vi "Editor UI.vi"(10 "Close Event":refnum<user-event>, 11 "Simulated Waveform in":refnum<class "Simulated Waveform.lvclass">) -> ()   [LabVIEW 2020, in "Simulated Waveform.lvlib" / "Simulated Waveform.lvclass"]
uses:
  Simulated Waveform.lvclass
  build/ppl/lv-hal.lvlibp/Device/Editor Event Data.ctl
  build/ppl/Signal Generator.lvlibp/Signal Generator/Waveform Type.ctl
  Simulated Waveform.lvclass/Simulated Waveform.ctl
  build/ppl/Signal Generator.lvlibp/Signal Generator/Waveform Definition.ctl
  build/ppl/Signal Generator.lvlibp/Signal Generator/Signal Generator.lvclass
  C:/dev/HAL Demo/build/ppl/Signal Generator.lvlibp/Signal Generator/Signal Generator.lvclass
  C:/dev/HAL Demo/build/ppl/lv-hal.lvlibp/Device/Device.lvclass
  build/ppl/lv-hal.lvlibp/Device/Device.lvclass
panel:
  in  "Sim Queue Name":string
  in  "Amplitude":dbl
  in  "Frequency":dbl
  in  "Waveform Type":T1
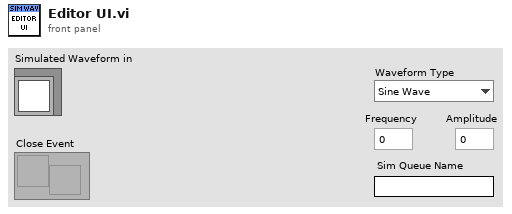
[diagram p1: front panel]
types:
  T1 = typedef "Signal Generator.lvlibp/Signal Generator.lvclass/Waveform Type.ctl" = enum16{"Sine Wave", "Triangle Wave", "Square Wave", "Sawtooth Wave"}
  T2 = typedef "Signal Generator.lvlibp/Signal Generator.lvclass/Waveform Definition.ctl" = cluster{"Waveform Type":T1, "Frequency":dbl, "Amplitude":dbl}
  T3 = typedef "Simulated Waveform.lvlib/Simulated Waveform.lvclass/Ref Data.ctl" = cluster{"Sim Queue Name":string, "Waveform Queue":refnum<queue>, "Noise Factor":dbl}
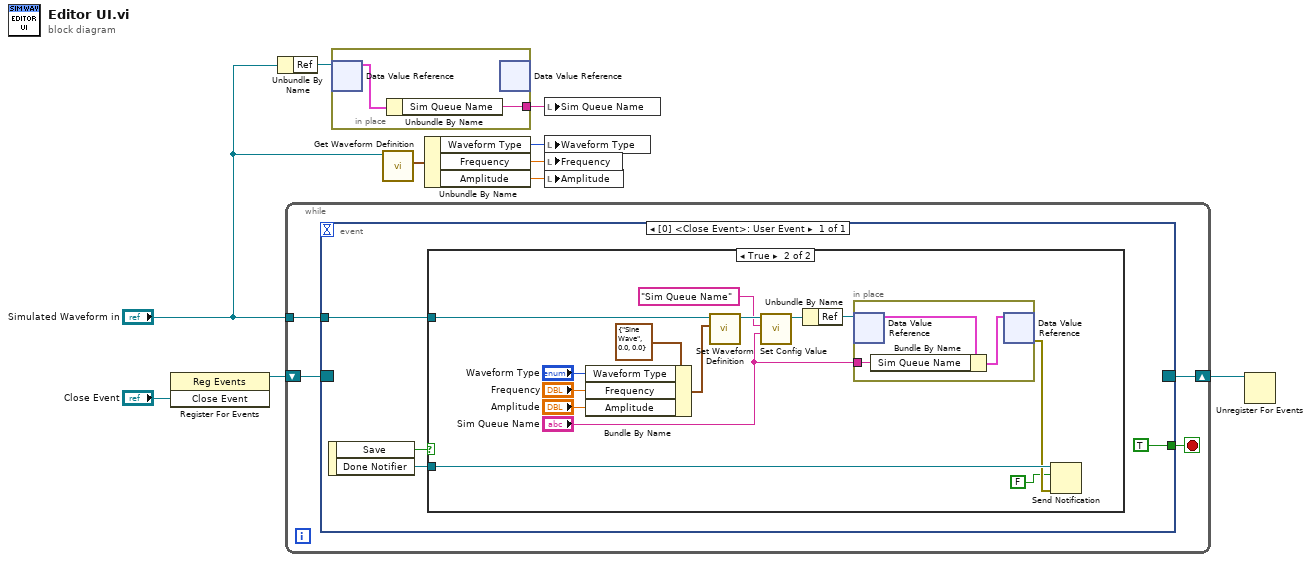
[diagram p0: block diagram]
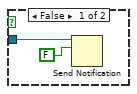
[diagram p2: hidden frame]
diagram:
  n1 = register-events("Close Event") -> (reference out=w9:refnum<event-registration>)  [unwired: 2 in, 1 out]
  n2 = Unbundle By Name("Simulated Waveform in") -> ("Ref"=w7:refnum<data-value>)
  n3 = while {
    shift-right: [w13] -> w8
    shift-left: w9 -> [w14]
    tunnel: "Simulated Waveform in" -> [w12]
    stop <- w11 stop-if-true
    n4 = event shown="[0] <Close Event>: User Event" {
      selector: w14 -> [_]
      dyn-events: [_] -> w13
      timeout: _ -> [_]
      tunnel: w12 -> [w16]
      tunnel: [TRUE] -> w11
      event User Event {
        n5 = event-data() -> ("Save"=w17:bool, "Done Notifier"=w18:refnum<notifier>)  [unwired: 1 in]
        n6 = case shown="True" w17 {
          tunnel: w18 -> [w20 w23]
          tunnel: w16 -> [_ w34]
          frame False {
            n7 = Send Notification(notification=FALSE, notifier=w20) -> ()  [unwired: 1 in, 2 out]
          }
          frame True {
            n8 = Bundle By Name(cluster=T2 {"Waveform Type"=enum."Sine Wave", "Frequency"=0.0, "Amplitude"=0.0} ("Waveform Definition"), "Waveform Type"="Waveform Type", "Frequency"="Frequency", "Amplitude"="Amplitude") -> (w32:T2)
            n9 = call "Set Waveform Definition.vi"("Waveform Definition"=w32, "Signal Generator in"=w34) -> ("Signal Generator out"=w28:refnum<class "Simulated Waveform.lvclass">)  [unwired: 8 in, 1 out]
            n10 = call "Set Config Value.vi"("Value"="Sim Queue Name", "Config Key"="Sim Queue Name", "Device in"=w28) -> ("Device out"=w25:refnum<class "Simulated Waveform.lvclass">)  [unwired: 7 in, 1 out]
            n11 = Unbundle By Name(w25) -> ("Ref"=w26:refnum<data-value>)
            n12 = in-place {
              in-place-border: "Sim Queue Name" -> [w35]
              n13 = in-place-dvr #1(w26) -> (w37:T3)  [unwired: 1 out]
              n14 = Bundle By Name(cluster=w37, "Sim Queue Name"=w35) -> (w36:T3)
              n15 = in-place-dvr #1(w36) -> (w22:errorcluster)  [unwired: 1 out]
            }
            n16 = Send Notification(notification=FALSE, notifier=w23, error in (no error)=w22) -> ()  [unwired: 2 out]
          }
        }
      }
    }
  }
  n17 = in-place {
    in-place-border: [w38] -> w5
    n18 = in-place-dvr #2(w7) -> (w39:T3)  [unwired: 1 out]
    n19 = Unbundle By Name(w39) -> ("Sim Queue Name"=w38:string)
    n20 = in-place-dvr #2() -> ()  [unwired: 1 in, 2 out]
  }
  n21 = call "Get Waveform Definition.vi"("Signal Generator in"="Simulated Waveform in") -> ("Waveform Definition"=w4:T2)  [unwired: 8 in, 2 out]
  n22 = Unbundle By Name(w4) -> ("Waveform Type"=w3:T1, "Frequency"=w2:dbl, "Amplitude"=w1:dbl)
  n23 = local write "Sim Queue Name"(w5) -> ()
  n24 = local write "Waveform Type"(w3) -> ()
  n25 = local write "Frequency"(w2) -> ()
  n26 = local write "Amplitude"(w1) -> ()
  n27 = Unregister For Events(event registration refnum=w8) -> ()  [unwired: 1 in, 1 out]
